vi "Simulation.vi"() -> (0 "output cluster":T1)   [LabVIEW 2019]
panel:
  out "Расходомер":dbl(slide) scale=0.1..5.0
  in  "Расходомер":dbl(slide) scale=0.1..5.0
  out "Манометр":dbl(slide) scale=3.0..6.0
  in  "Манометр":dbl(slide) scale=3.0..6.0
  out "ДМ2-вывод":dbl(slide) scale=0.0..200.0
  in  "ДМ2":dbl(slide) scale=0.0..200.0
  out "ДМ1-вывод":dbl(slide) scale=0.0..14.0
  in  "ДМ1":dbl(slide) scale=0.0..14.0
  out "PH1-вывод":dbl(slide) scale=0.0..14.0
  in  "PH1":dbl(slide) scale=0.0..14.0
  out "УЗ7-вывод":dbl(slide) scale=0.0..100.0
  in  "УЗ7":dbl(slide) min=0.0 max=100.0 step=1.0 scale=0.0..100.0
  out "УЗ6-вывод":dbl(slide) scale=0.0..100.0
  in  "УЗ6":dbl(slide) min=0.0 max=100.0 step=1.0 scale=0.0..100.0
  out "УЗ5-вывод":dbl(slide) scale=0.0..100.0
  in  "УЗ5":dbl(slide) min=0.0 max=100.0 step=1.0 scale=0.0..100.0
  out "УЗ4-вывод":dbl(slide) scale=0.0..100.0
  in  "УЗ4":dbl(slide) min=0.0 max=100.0 step=1.0 scale=0.0..100.0
  out "УЗ3-вывод":dbl(slide) scale=0.0..100.0
  in  "УЗ3":dbl(slide) min=0.0 max=100.0 step=1.0 scale=0.0..100.0
  out "УЗ2-вывод":dbl(slide) scale=0.0..100.0
  in  "УЗ2":dbl(slide) min=0.0 max=100.0 step=1.0 scale=0.0..100.0
  out "УЗ1-вывод":dbl(slide) scale=0.0..100.0
  in  "УЗ1":dbl(slide) min=0.0 max=100.0 step=1.0 scale=0.0..100.0
  # "Симуляция показаний датчиков"
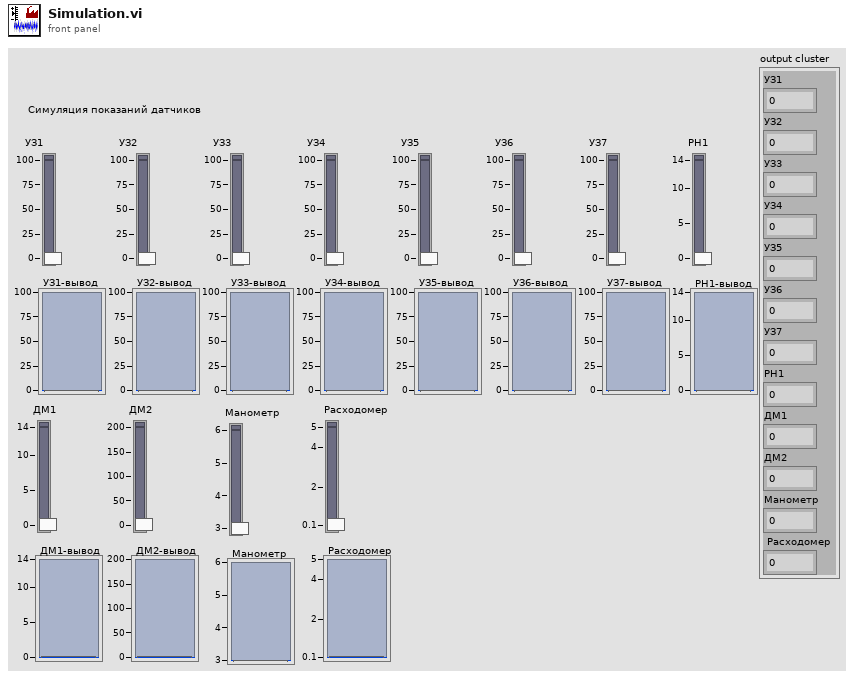
[diagram p1: front panel]
types:
  T1 = cluster{"УЗ1":dbl, "УЗ2":dbl, "УЗ3":dbl, "УЗ4":dbl, "УЗ5":dbl, "УЗ6":dbl, "УЗ7":dbl, "PH1":dbl, "ДМ1":dbl, "ДМ2":dbl, "Манометр":dbl, " Расходомер":dbl}
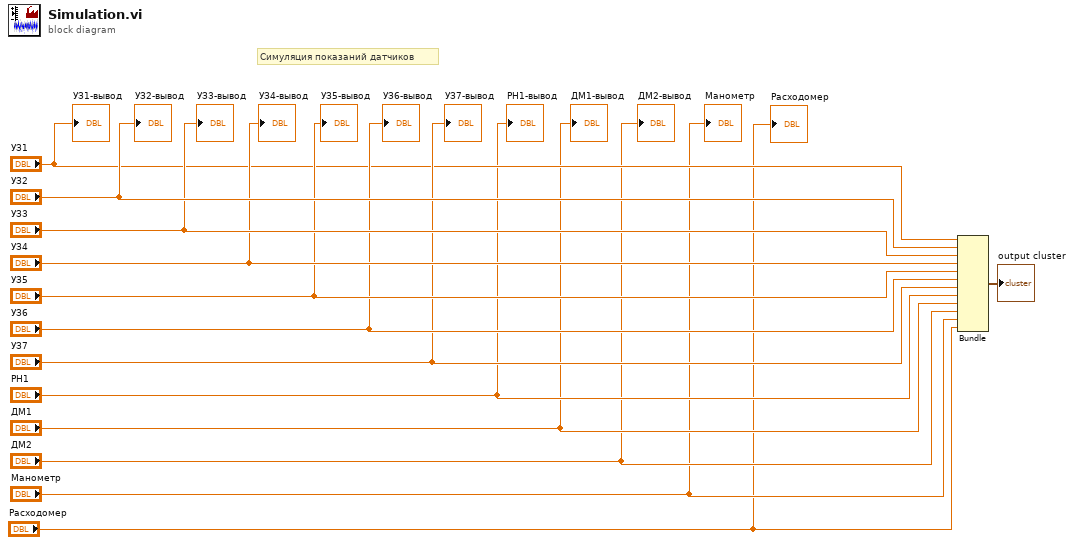
[diagram p0: block diagram]
diagram:
  # "Симуляция показаний датчиков"
  n1 = Bundle("УЗ1"="УЗ1", "УЗ2"="УЗ2", "УЗ3"="УЗ3", "УЗ4"="УЗ4", "УЗ5"="УЗ5", "УЗ6"="УЗ6", "УЗ7"="УЗ7", "PH1"="PH1", "ДМ1"="ДМ1", "ДМ2"="ДМ2", "Манометр"="Манометр", "Расходомер"="Расходомер") -> (→"output cluster":T1)  [unwired: 1 in]
  "УЗ1-вывод" <- "УЗ1"
  "УЗ2-вывод" <- "УЗ2"
  "УЗ3-вывод" <- "УЗ3"
  "УЗ4-вывод" <- "УЗ4"
  "УЗ5-вывод" <- "УЗ5"
  "УЗ6-вывод" <- "УЗ6"
  "УЗ7-вывод" <- "УЗ7"
  "PH1-вывод" <- "PH1"
  "ДМ1-вывод" <- "ДМ1"
  "ДМ2-вывод" <- "ДМ2"
  "Манометр" <- "Манометр"
  "Расходомер" <- "Расходомер"
